vi "Parse.vi"(8 "Error In":errorcluster, 11 "object in":refnum<class "2022_1.lvclass">) -> (0 "Error Out":errorcluster, 3 "object out":refnum<class "2022_1.lvclass">)   [LabVIEW 2020, in "2022_1.lvclass"]
uses:
  2022_1.lvclass
  2022_1.lvclass/2022_1.ctl
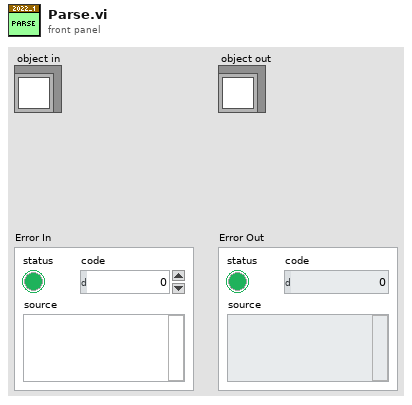
[diagram p1: front panel]
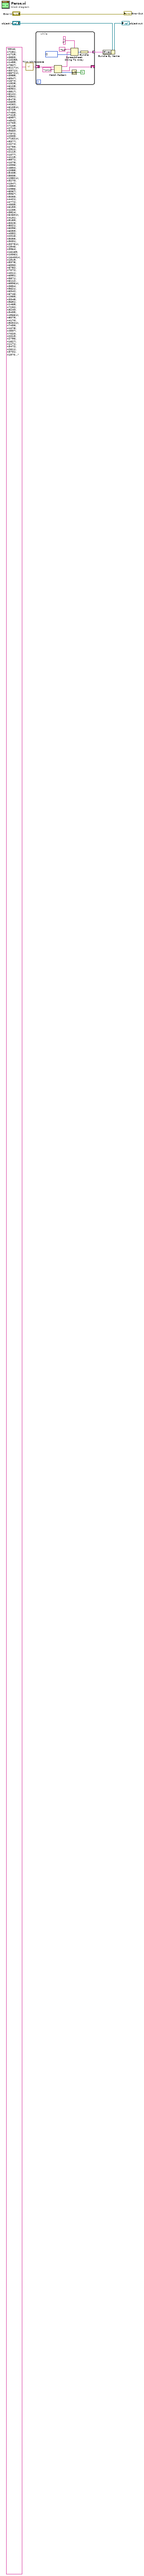
[diagram p0: block diagram]
diagram:
  n1 = call <vilib>:"Trim Whitespace.vi"("string"="5916\n7281\n1715\n3853\n10283\n1455\n7807\n6117\n\n33711\n6672\n\n3988\n6947\n1674\n1928\n6128\n6361\n3817\n6141\n3301\n5473\n2609\n4262\n6105\n\n2725\n7430\n7415\n6997\n4542\n2703\n7148\n2710\n5660\n7372\n2539\n7162\n\n5377\n4274\n2793\n2911\n2113\n1077\n4115\n5871\n1079\n4336\n4894\n2088\n5408\n5535\n1982\n\n3270\n1347\n4884\n2986\n6067\n5567\n5093\n4421\n2772\n4935\n6153\n1235\n3824\n6460\n\n4131\n5183\n5329\n8021\n6096\n6053\n4352\n2016\n5055\n3031\n3379\n\n1846\n3964\n16169\n10061\n16400\n\n1519\n5378\n6590\n6782\n7072\n4011\n6581\n5871\n6112\n6836\n\n3894\n5621\n6342\n6746\n1955\n3348\n5651\n1468\n7232\n3240\n3435\n4566\n\n8079\n4170\n5034\n\n7439\n1078\n4537\n7020\n2013\n2796\n1627\n1171\n3472\n2611\n3701\n1570..." ("PuzzleInput")) -> ("trimmed string"=w1:string)  [unwired: 1 in]
  n2 = while {
    shift-right: [w15] -> _
    shift-left: w1 -> [w17]
    tunnel: [w7] -> w2 mode=indexing
    stop <- w13 continue-if-true
    n3 = Match Pattern(string=w17, regular expression="\\n\\n") -> (before substring=w9:string, after substring=w15:string, offset past match=w14:i32)  [unwired: 1 in, 1 out]
    n4 = Greater Or Equal To 0?(x=w14) -> (x >= 0?=w13:bool)
    n5 = Spreadsheet String To Array(delimiter (Tab)="\n", format string="%d", spreadsheet string=w9, array type (2D Dbl)=u64[] []) -> (array=w8:u64[])
    n6 = Bundle("array type (2D Dbl)"=w8) -> (w7:cluster{"array type (2D Dbl)":u64[]})  [unwired: 1 in]
  }
  n7 = Bundle By Name(cluster="object in", "Elves"=w2) -> (→"object out":refnum<class "2022_1.lvclass">)
  "Error Out" <- "Error In"
